vi "Abort.vi"(8 "error in (no error)":errorcluster, 11 "PI650 VoltageAmp in":refnum<class "PI650 VoltageAmp.lvclass">) -> (0 "error out":errorcluster, 3 "PI650 VoltageAmp out":refnum<class "PI650 VoltageAmp.lvclass">)   [LabVIEW 2020, in "Pickering.lvlib" / "PI650 VoltageAmp.lvclass"]
uses:
  PI650 VoltageAmp.lvclass
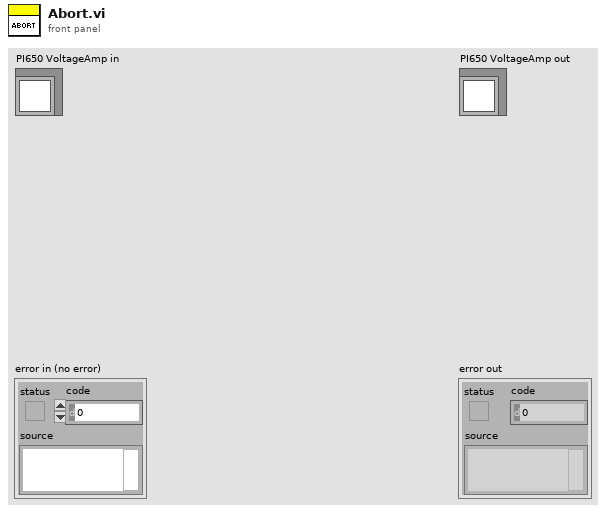
[diagram p1: front panel]
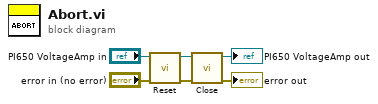
[diagram p0: block diagram]
diagram:
  n1 = call-dynamic "Reset.vi"("error in (no error)"="error in (no error)", "PI650 VoltageAmp in"="PI650 VoltageAmp in") -> ("error out"=w6:errorcluster, "PI650 VoltageAmp out"=w5:refnum<class "PI650 VoltageAmp.lvclass">)  [unwired: 8 in]
  n2 = call-dynamic "Close.vi"("error in (no error)"=w6, "PI650 VoltageAmp in"=w5) -> ("error out"=→"error out":errorcluster, "PI650 VoltageAmp out"=→"PI650 VoltageAmp out":refnum<class "PI650 VoltageAmp.lvclass">)  [unwired: 8 in]
